vi "Drive Activate.vi"(9 "Right Joystick":dbl, 11 "Left Joystick":dbl) -> ()   [LabVIEW 2012]
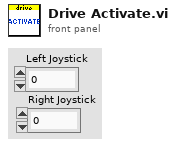
[diagram p1: front panel]
types:
  T1 = typedef "WPI_MotorControlDeviceRef.ctl" = cluster{"DeviceStatus":errorcluster, "Type":enum16{"PWM", "CAN"}, "PWM":cluster{"Digital Module":T2, "PWM Channel":T3, "DeadBand":T4}, "CAN":cluster{"Device Number":u8, "Control Mode":T5, "Semaphore":T6, "Max Vout":dbl}, "Invert":bool, "TransformRef":T7, "InvTransformRef":T7}
  T2 = typedef "FPGA_TypedefDigitalModule.ctl" = enum16{"Digital Module 1", "Digital Module 2"}
  T3 = typedef "FPGA_DIOPWMChannel.ctl" = enum8{"PWM 1", "PWM 2", "PWM 3", "PWM 4", "PWM 5", "PWM 6", "PWM 7", "PWM 8", "PWM 9", "PWM 10", "Invalid"}
  T4 = typedef "WPI_PWMDeadband.ctl" = cluster{"Name":string, "maxPositivePwm":i32, "minPositivePwm":i32, "centerPwm":i32, "maxNegativePwm":i32, "minNegativePwm":i32, "angularRange":u16}
  T5 = typedef "WPI_CANJaguar_ControlMode.ctl" = enum8{"Percent VBus", "Current", "Speed", "Position", "Voltage"}
  T6 = typedef "Semaphore RefNum" = refnum<k1>
  T7 = typedef "WPI_PWMTransform_ConPane.ctl" = refnum<vi>
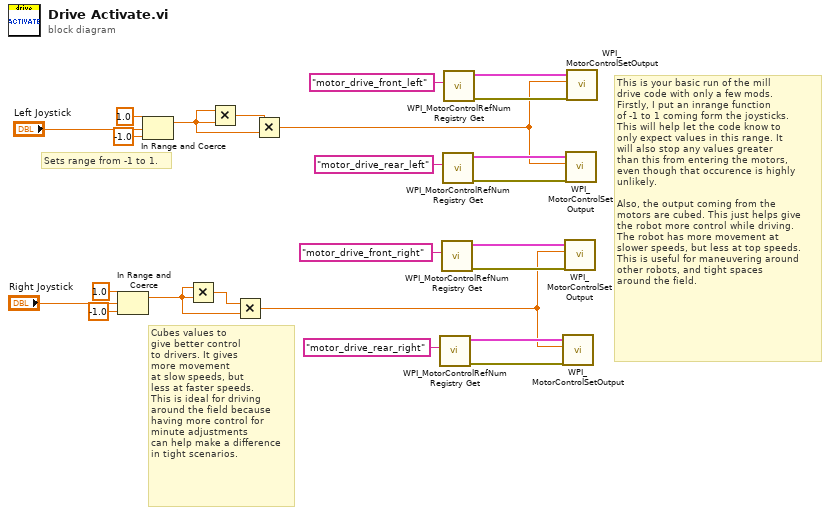
[diagram p0: block diagram]
diagram:
  # "This is your basic run of the mill\ndrive code with only a few mods. \nFirstly, I put an inrange function \nof -1 to 1 coming form the joysticks.\nThis will help let the code know to \nonly expect values in this range. It\nwill also stop any values greater \nthan this from entering the motors, \neven though that occurence is highly\nunlikely. \n\nAlso, the output coming from the \nmotors are cubed. This just helps give \nthe robot more control while driving. \nThe robot has more movement at\nslower speeds, but less at top speeds. \nThis is useful for maneuvering around \nother robots, and tight spaces\naround the field."
  # "Cubes values to \ngive better control\nto drivers. It gives\nmore movement\nat slow speeds, but \nless at faster speeds.\nThis is ideal for driving\naround the field because\nhaving more control for\nminute adjustments\ncan help make a difference\nin tight scenarios."
  # "Sets range from -1 to 1."
  n1 = In Range and Coerce(upper limit=1.0, x="Right Joystick", lower limit=-1.0) -> (coerced(x)=w2:dbl)  [unwired: 1 out]
  n2 = In Range and Coerce(upper limit=1.0, x="Left Joystick", lower limit=-1.0) -> (coerced(x)=w5:dbl)  [unwired: 1 out]
  n3 = Multiply(x=w2, y=w2) -> (x*y=w3:dbl)
  n4 = Multiply(x=w5, y=w5) -> (x*y=w6:dbl)
  n5 = Multiply(x=w3, y=w2) -> (x*y=w1:dbl)
  n6 = Multiply(x=w6, y=w5) -> (x*y=w4:dbl)
  n7 = call <vilib>:"WPI_MotorControlRefNum Registry Get.vi"("refnum name"="motor_drive_rear_right") -> ("error out"=w18:errorcluster, "MotorControlDevRef"=w17:T1)  [unwired: 9 in]
  n8 = call <vilib>:"WPI_MotorControlRefNum Registry Get.vi"("refnum name"="motor_drive_front_right") -> ("error out"=w19:errorcluster, "MotorControlDevRef"=w20:T1)  [unwired: 9 in]
  n9 = call <vilib>:"WPI_MotorControlRefNum Registry Get.vi"("refnum name"="motor_drive_rear_left") -> ("error out"=w22:errorcluster, "MotorControlDevRef"=w21:T1)  [unwired: 9 in]
  n10 = call <vilib>:"WPI_MotorControlRefNum Registry Get.vi"("refnum name"="motor_drive_front_left") -> ("error out"=w23:errorcluster, "MotorControlDevRef"=w24:T1)  [unwired: 9 in]
  n11 = call <vilib>:"WPI_MotorControlSetOutput.vi"("error in (no error)"=w18, "Output"=w1, "MotorControlDevRef"=w17) -> ()  [unwired: 6 in, 3 out]
  n12 = call <vilib>:"WPI_MotorControlSetOutput.vi"("error in (no error)"=w19, "Output"=w1, "MotorControlDevRef"=w20) -> ()  [unwired: 6 in, 3 out]
  n13 = call <vilib>:"WPI_MotorControlSetOutput.vi"("error in (no error)"=w22, "Output"=w4, "MotorControlDevRef"=w21) -> ()  [unwired: 6 in, 3 out]
  n14 = call <vilib>:"WPI_MotorControlSetOutput.vi"("error in (no error)"=w23, "Output"=w4, "MotorControlDevRef"=w24) -> ()  [unwired: 6 in, 3 out]
